vi "Get VI Reference.vi"(8 "error in (no error)":errorcluster, 11 "VI Name":string) -> (0 "error out":errorcluster, 3 "VI Ref":refnum<vi>)   [LabVIEW 2020, in "MacroAssert.lvlib"]
uses:
  MacroAssert.lvlib
  CTLs/FGV Actions.ctl
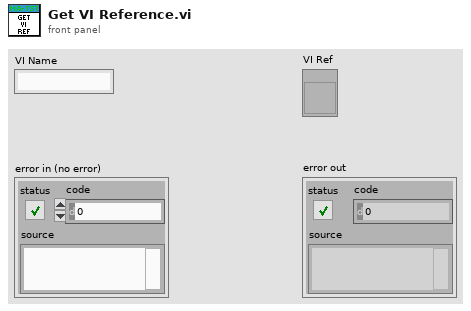
[diagram p1: front panel]
types:
  T1 = typedef "MacroAssert.lvlib/FGV Actions.ctl" = enum16{"Read", "Write"}
  T2 = enum32{"invalid app kind", "Development System", "Run Time System", "Student Edition", "Embedded LabVIEW", "Evaluation", "Custom"}
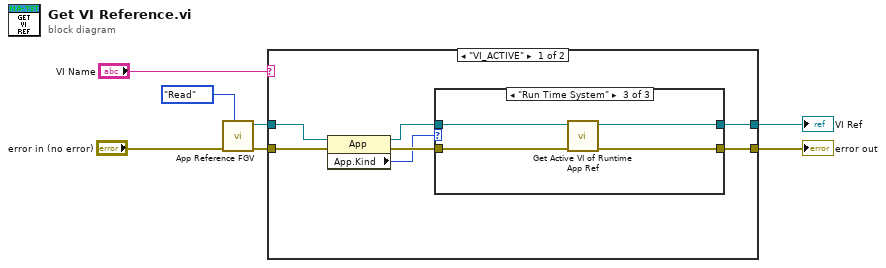
[diagram p0: block diagram]
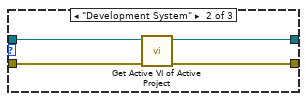
[diagram p3: hidden frame]
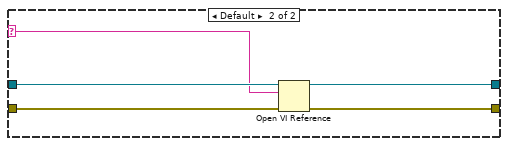
[diagram p4: hidden frame]
diagram:
  n1 = call "App Reference FGV.vi"("Mode"=FGV_Actions."Read", "error in (no error)"="error in (no error)") -> ("error out"=w6:errorcluster, "App Ref out"=w3:refnum<vi>)  [unwired: 8 in]
  n2 = case shown="\"VI_ACTIVE\"" "VI Name" {
    selector: "VI Name" -> [_ w24]
    tunnel: [w14 w28] -> w7
    tunnel: [w13 w26] -> w4
    tunnel: w3 -> [w12 w25]
    tunnel: w6 -> [w11 w27]
    frame "VI_ACTIVE" {
      n3 = property class="App"(reference=w12, error in=w11) -> (reference out=w10:refnum<vi>, error out=w9:errorcluster, "App.Kind"=w8:T2)
      n4 = case shown="\"Run Time System\"" w8 {
        tunnel: w9 -> [w15 w19 w23]
        tunnel: [w15 w18 w22] -> w14
        tunnel: [_ w17 w21] -> w13
        tunnel: w10 -> [_ w16 w20]
        frame "invalid app kind", Default {
          # "#TODO custom error"
        }
        frame "Development System" {
          n5 = call "Get Active VI of Active Project.vi"("error in (no error)"=w19, "App Ref"=w16) -> ("error out"=w18:errorcluster, "Active VI Ref"=w17:refnum<vi>)  [unwired: 8 in]
        }
        frame "Run Time System" {
          n6 = call "Get Active VI of Runtime App Ref.vi"("error in (no error)"=w23, "App Ref"=w20) -> ("error out"=w22:errorcluster, "Active VI Ref"=w21:refnum<vi>)  [unwired: 8 in]
        }
      }
    }
    frame Default {
      n7 = Open VI Reference(application reference (local)=w25, vi path=w24, error in (no error)=w27) -> (vi reference=w26:refnum<vi>, error out=w28:errorcluster)  [unwired: 3 in]
    }
  }
  "error out" <- w7
  "VI Ref" <- w4
